vi "MCLB_MouseDown.vi"(8 "error in":errorcluster, 9 "Coords":T1, 10 "Button":u16, 11 "MCListbox Refnum":refnum<vi>) -> (0 "error out":errorcluster)   [LabVIEW 2014]
doc: "Changes clicked item symbol to 'select/unselect symbol'"
uses:
  <vilib>/Utility/miscctls.llb/LVPoint32TypeDef.ctl
panel:
  in  "Single Select? (F)":bool
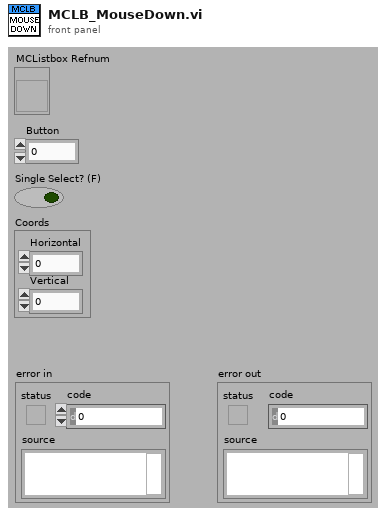
[diagram p1: front panel]
types:
  T1 = typedef "LVPoint32TypeDef.ctl" = cluster{"Horizontal":i32, "Vertical":i32}
  T2 = typedef "LVRowAndColumnTypeDef.ctl" = cluster{"Row":i32, "Column":i32}
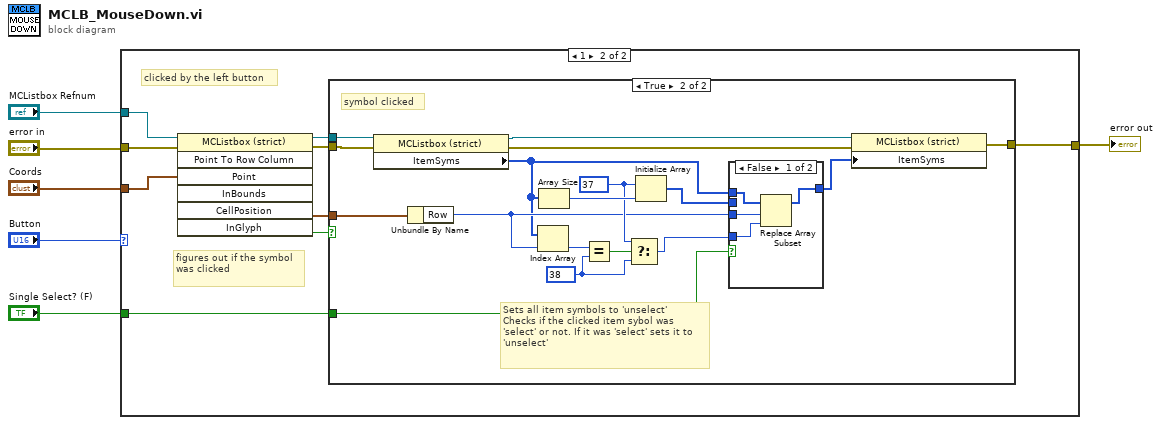
[diagram p0: block diagram]
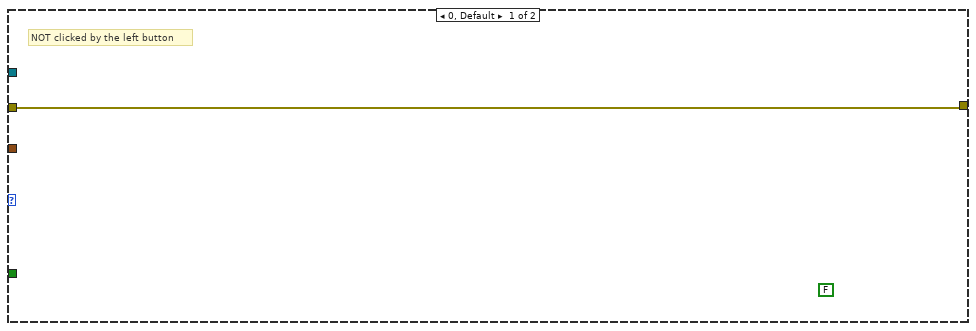
[diagram p2: hidden frame]
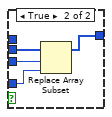
[diagram p4: hidden frame]
diagram:
  n1 = case shown="1" "Button" {
    tunnel: "Coords" -> [_ w16]
    tunnel: "error in" -> [w7 w12]
    tunnel: [w7 w11] -> w5
    tunnel: "MCListbox Refnum" -> [_ w10]
    tunnel: "Single Select? (F)" -> [_ w8]
    frame 0, Default {
      (unwired) FALSE
      # "NOT clicked by the left button"
    }
    frame 1 {
      # "clicked by the left button"
      # "figures out if the symbol was clicked"
      n2 = invoke on="Invoke Node" class="MCListbox (strict)" method="Point To Row Column"(reference=w10, error in=w12, "Point"=w16) -> (reference out=w9:refnum<vi>, error out=w13:errorcluster, "CellPosition"=w15:T2, "InGlyph"=w14:bool)  [unwired: 4 in, 3 out]
      n3 = case shown="True" w14 {
        tunnel: w15 -> [_ w34]
        tunnel: w13 -> [w17 w33]
        tunnel: [w17 w28] -> w11
        tunnel: w9 -> [_ w27]
        tunnel: w8 -> [_ w19]
        frame False {
          # "symbol NOT clicked"
        }
        frame True {
          w22 = 38
          w23 = 37
          # "symbol clicked"
          # "Sets all item symbols to 'unselect'\nChecks if the clicked item sybol was 'select' or not. If it was 'select' sets it to 'unselect'"
          n4 = property on="Property Node" class="MCListbox (strict)"(reference=w27, error in=w33) -> (reference out=w26:refnum<vi>, error out=w32:errorcluster, "ItemSyms"=w18:i32[])
          n5 = Unbundle By Name(w34) -> ("Row"=w20:i32)
          n6 = Index Array(array=w18, index=w20) -> (element=w25:i32)
          n7 = Array Size(array=w18) -> (size(s)=w29:i32)
          n8 = Equal?(x=w25, y=w22) -> (x = y?=w24:bool)
          n9 = Select(t=w23, s=w24, f=w22) -> (s? t:f=w21:i32)
          n10 = Initialize Array(w23, w29) -> (w31:i32[])
          n11 = case shown="False" w19 {
            tunnel: w31 -> [_ w42]
            tunnel: [w37 w41] -> w30
            tunnel: w21 -> [w38 w40]
            tunnel: w20 -> [w36 w39]
            tunnel: w18 -> [w35 _]
            frame False {
              n12 = Replace Array Subset(array=w35, new element=w38, index=w36) -> (w37:i32[])
            }
            frame True {
              n13 = Replace Array Subset(array=w42, new element=w40, index=w39) -> (w41:i32[])
            }
          }
          n14 = property on="Property Node" class="MCListbox (strict)"(reference=w26, error in=w32, "ItemSyms"=w30) -> (error out=w28:errorcluster)  [unwired: 1 out]
        }
      }
    }
  }
  "error out" <- w5
